vi "Read Data.vi"(8 "error in (no error)":errorcluster, 11 "Keithley Source in":refnum<class "Keithley Source.lvclass">) -> (0 "error out":errorcluster, 2 "Data":waveform(dbl)[](array[waveform]), 3 "Keithley Source out":refnum<class "Keithley Source.lvclass">)   [LabVIEW 2015, in "Keithley Source.lvclass"]
uses:
  Keithley Source.lvclass
  Keithley Source.lvclass/Keithley Source.ctl
  Instrument/Read VISA Resource.vi
  Instrument/Write VISA Resource.vi
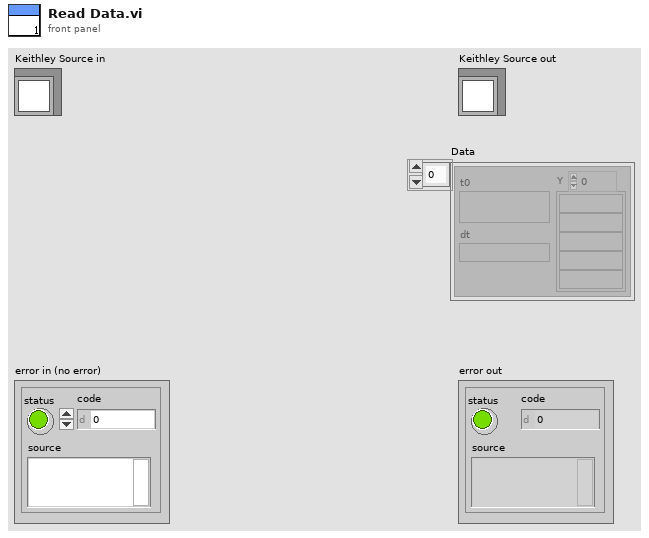
[diagram p1: front panel]
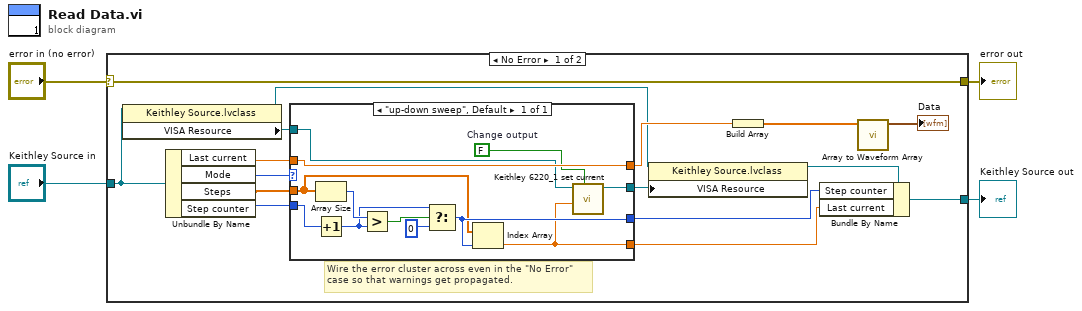
[diagram p0: block diagram]
diagram:
  n1 = case shown="No Error" "error in (no error)" {
    selector: "error in (no error)" -> [w20 w34]
    tunnel: [w20 w34] -> w3
    tunnel: [w11 w33] -> w1
    tunnel: "Keithley Source in" -> [w19 w33]
    frame No Error {
      # "Wire the error cluster across even in the \"No Error\"\ncase so that warnings get propagated."
      n2 = property class="Keithley Source.lvclass"(reference=w19) -> (reference out=w8:refnum<class "Keithley Source.lvclass">, "VISA Resource"=w7:refnum<visa-resource-name>)  [unwired: 1 in, 1 out]
      n3 = Unbundle By Name(w19) -> ("Last current"=w15:dbl, "Mode"=w18:enum16{"up-down sweep"}, "Steps"=w16:dbl[], "Step counter"=w17:i32)
      n4 = case shown="\"up-down sweep\", Default" w18 {
        tunnel: w17 -> [w32]
        tunnel: w16 -> [w25]
        tunnel: w15 -> [w27]
        tunnel: [w27] -> w12
        tunnel: [w26] -> w10
        tunnel: [w24] -> w9
        tunnel: w7 -> [w22]
        tunnel: [w21] -> w5
        frame "up-down sweep", Default {
          w23 = FALSE  # Change output
          n5 = Array Size(array=w25) -> (size(s)=w31:i32)
          n6 = Increment(x=w32) -> (x+1=w29:i32)
          n7 = Greater?(x=w31, y=w29) -> (0:w30:bool)
          n8 = Select(t=w29, s=w30, f=0) -> (s? t:f=w26:i32)
          n9 = Index Array(array=w25, index=w26) -> (element=w24:dbl)
          n10 = call "Keithley 6220_1 set current.vi"("Change output"=w23, "Current (A)"=w24, "VISA resource name"=w22) -> ("VISA resource name out"=w21:refnum<visa-resource-name>)  [unwired: 7 in, 1 out]
        }
      }
      n11 = property class="Keithley Source.lvclass"(reference=w8, "VISA Resource"=w5) -> (reference out=w6:refnum<class "Keithley Source.lvclass">)  [unwired: 1 in, 1 out]
      n12 = Build Array(w12) -> (w13:dbl[])
      n13 = Bundle By Name(cluster=w6, "Step counter"=w10, "Last current"=w9) -> (w11:refnum<class "Keithley Source.lvclass">)
      n14 = call "Array to Waveform Array.vi"("Array"=w13) -> ("Waveform"=→"Data":waveform(dbl)[])  [unwired: 10 in]
    }
    frame Error {
    }
  }
  "error out" <- w3
  "Keithley Source out" <- w1
